vi "Decode Message.vi"(8 "Error In":errorcluster, 11 "Image 2 Path in":path) -> (0 "Error Out":errorcluster, 3 "Decoded Message":string)   [LabVIEW 2020]
uses:
  <vilib>/Utility/libraryn.llb/Generate Temporary File Path.vi
  <vilib>/zip/Unzip.vi
  <vilib>/Utility/file.llb/Application Directory.vi
  <vilib>/Platform/system.llb/System Exec.vi
  Image Comparison/Image Comparison.lvclass
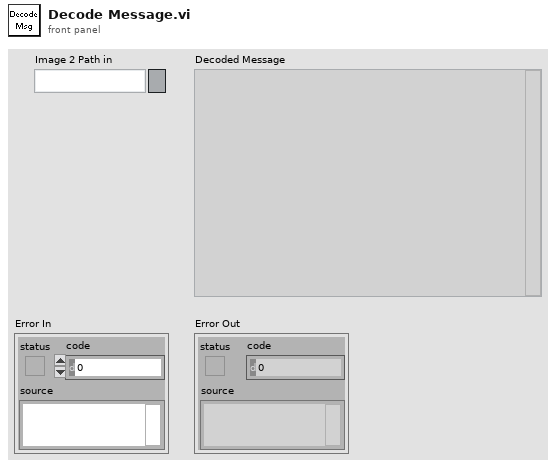
[diagram p1: front panel]
types:
  T1 = typedef "imagedata.ctl" = cluster{"image type":i32, "image depth":i32, "image":u8[], "mask":u8[], "colors":u32[], "Rectangle":cluster{"left":i16, "top":i16, "right":i16, "bottom":i16}}
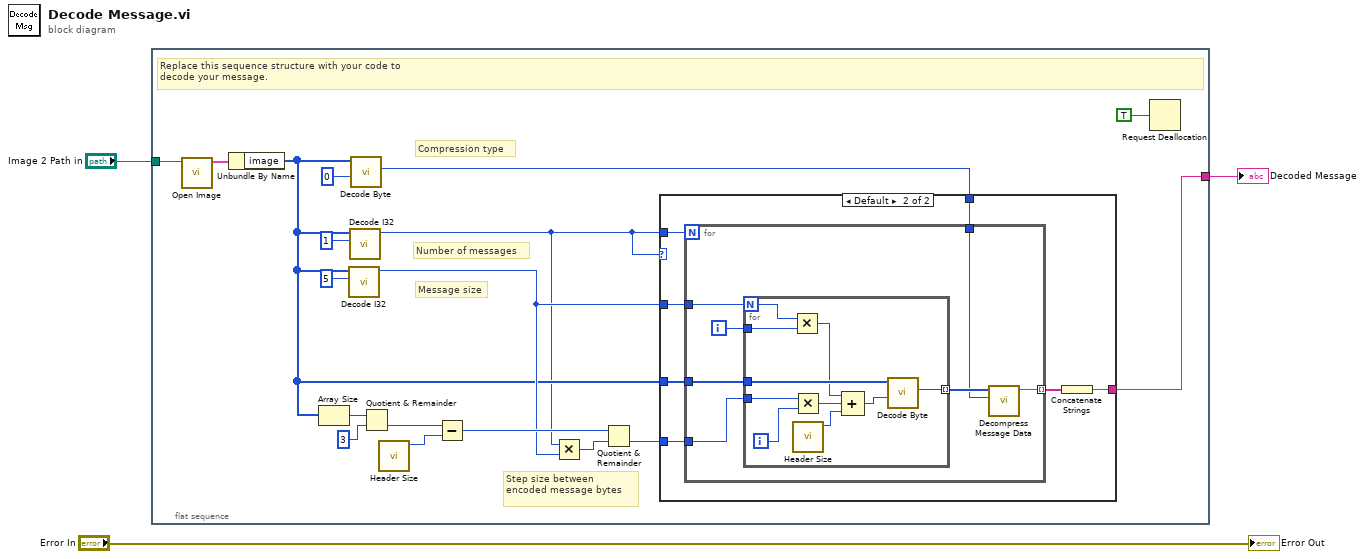
[diagram p0: block diagram]
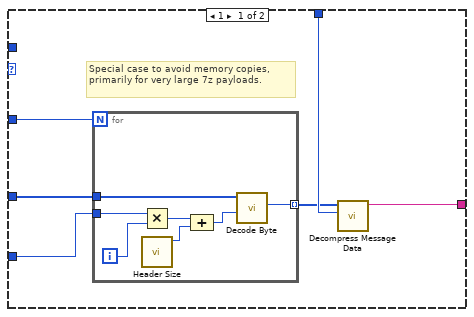
[diagram p2: hidden frame]
diagram:
  n1 = flat-sequence {
    tunnel: "Image 2 Path in" -> [w21]
    tunnel: [w11] -> w1
    frame #0 {
      # "Compression type"
      # "Step size between encoded message bytes"
      # "Message size"
      # "Number of messages"
      # "Replace this sequence structure with your code to \ndecode your message."
      n2 = call "Open Image.vi"("Image"=w21) -> ("image data"=w20:T1)  [unwired: 9 in, 1 out]
      n3 = Unbundle By Name(w20) -> ("image"=w9:u8[])
      n4 = Array Size(array=w9) -> (size(s)=w16:i32)
      n5 = call "Decode I32.vi"("Pixel Offset (0)"=5, "Image In"=w9) -> ("I32"=w12:i32)  [unwired: 9 in]
      n6 = call "Decode I32.vi"("Pixel Offset (0)"=1, "Image In"=w9) -> ("I32"=w4:i32)  [unwired: 9 in]
      n7 = call "Decode Byte.vi"("Pixel Offset"=0, "Image In"=w9) -> ("Decoded Byte"=w6:u8)  [unwired: 9 in]
      n8 = Quotient & Remainder(x=w16, y=3) -> (floor(x/y)=w14:i32)  [unwired: 1 out]
      n9 = call "Header Size.vi"() -> ("Header Size"=w5:i32)  [unwired: 11 in]
      n10 = Subtract(x=w14, y=w5) -> (x-y=w19:i32)
      n11 = Multiply(x=w4, y=w12) -> (x*y=w18:i32)
      n12 = Quotient & Remainder(x=w19, y=w18) -> (floor(x/y)=w17:i32)  [unwired: 1 out]
      n13 = case shown="Default" w4 {
        tunnel: w17 -> [w27 w41]
        tunnel: w4 -> [_ w40]
        tunnel: w12 -> [w26 w39]
        tunnel: [w22 w38] -> w11
        tunnel: w9 -> [w25 w36]
        tunnel: w6 -> [w24 w35]
        frame 1 {
          # "Special case to avoid memory copies, primarily for very large 7z payloads."
          n14 = for {
            N: w26 -> [_]
            tunnel: w25 -> [w34]
            tunnel: [w32] -> w23 mode=indexing
            tunnel: w27 -> [w31]
            i -> [w30]
            n15 = Multiply(x=w31, y=w30) -> (x*y=w29:i32)
            n16 = call "Header Size.vi"() -> ("Header Size"=w28:i32)  [unwired: 11 in]
            n17 = Compound Arithmetic op=ADD(w29, w28) -> (w33:i32)
            n18 = call "Decode Byte.vi"("Pixel Offset"=w33, "Image In"=w34) -> ("Decoded Byte"=w32:u8)  [unwired: 9 in]
          }
          n19 = call "Decompress Message Data.vi"("Compression (zip)"=w24, "Compressed Message"=w23) -> ("Message"=w22:string)  [unwired: 9 in]
        }
        frame Default {
          n20 = for {
            N: w40 -> [_]
            tunnel: w39 -> [w48]
            tunnel: w36 -> [w47]
            tunnel: w41 -> [w44]
            tunnel: [w43] -> w37 mode=indexing
            tunnel: w35 -> [w42]
            i -> [w46]
            n21 = for {
              N: w48 -> [w56]
              tunnel: w47 -> [w58]
              tunnel: w46 -> [w57]
              tunnel: [w53] -> w45 mode=indexing
              tunnel: w44 -> [w52]
              i -> [w51]
              n22 = Multiply(x=w56, y=w57) -> (x*y=w55:i32)
              n23 = Multiply(x=w52, y=w51) -> (x*y=w50:i32)
              n24 = call "Header Size.vi"() -> ("Header Size"=w49:i32)  [unwired: 11 in]
              n25 = Compound Arithmetic op=ADD(w55, w50, w49) -> (w54:i32)
              n26 = call "Decode Byte.vi"("Pixel Offset"=w54, "Image In"=w58) -> ("Decoded Byte"=w53:u8)  [unwired: 9 in]
            }
            n27 = call "Decompress Message Data.vi"("Compression (zip)"=w42, "Compressed Message"=w45) -> ("Message"=w43:string)  [unwired: 9 in]
          }
          n28 = Concatenate Strings(w37) -> (w38:string)
        }
      }
      n29 = Request Deallocation(TRUE ("flag")) -> ()
    }
  }
  "Error Out" <- "Error In"
  "Decoded Message" <- w1
